vi "OEE_SCREEN_2_map_over_cycle_time_record_to_cluster.vi"(11 "stations_over_cycle_time":i32[](array[numeric])) -> (1 "actual":string, 2 "target":string, 3 "station":string)   [LabVIEW 2019]
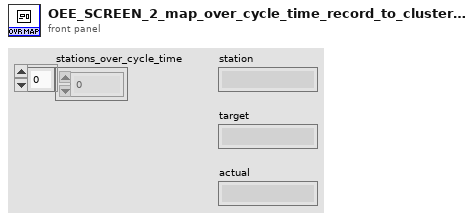
[diagram p1: front panel]
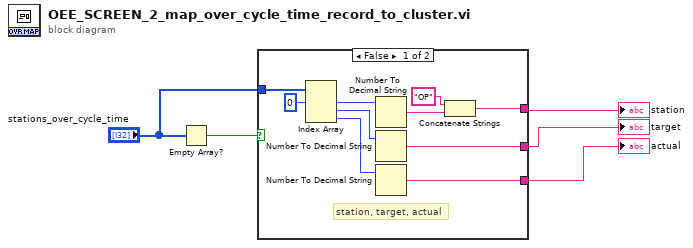
[diagram p0: block diagram]
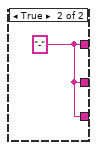
[diagram p2: hidden frame]
diagram:
  n1 = Empty Array?(array="stations_over_cycle_time") -> (empty?=w2:bool)
  n2 = case shown="False" w2 {
    tunnel: "stations_over_cycle_time" -> [w15 _]
    tunnel: [w8 w16] -> w3
    tunnel: [w7 w16] -> w4
    tunnel: [w6 w16] -> w5
    frame False {
      # "station, target, actual"
      n3 = Index Array(array=w15, index #1=0 ("index")) -> (element #1=w13:i32, element #2=w12:i32, element #3=w11:i32)  [unwired: 2 in]
      n4 = Number To Decimal String(number=w13) -> (decimal integer string=w10:string)  [unwired: 1 in]
      n5 = Number To Decimal String(number=w12) -> (decimal integer string=w7:string)  [unwired: 1 in]
      n6 = Number To Decimal String(number=w11) -> (decimal integer string=w6:string)  [unwired: 1 in]
      n7 = Concatenate Strings("OP" ("string"), w10) -> (w8:string)
    }
    frame True {
      w16 = "-"
    }
  }
  "actual" <- w5
  "target" <- w4
  "station" <- w3
